vi "TBQ_SetMaximumAge.vi"(9 "Maximum Age (s)":dbl, 11 "TimeBasedQueue In":refnum<class "TimeBasedQueue.lvclass">) -> (3 "TimeBasedQueue Out":refnum<class "TimeBasedQueue.lvclass">)   [LabVIEW 2012, in "TimeBasedQueue.lvclass"]
uses:
  TimeBasedQueue.lvclass
  TimeBasedQueue.lvclass/TimeBasedQueue.ctl
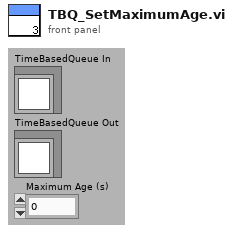
[diagram p1: front panel]
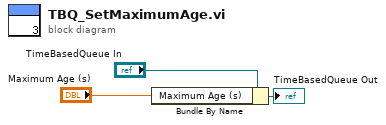
[diagram p0: block diagram]
diagram:
  n1 = Bundle By Name(cluster="TimeBasedQueue In", "Maximum Age (s)"="Maximum Age (s)") -> (→"TimeBasedQueue Out":refnum<class "TimeBasedQueue.lvclass">)
